vi "macro_MecaDrivePoseEst2_Execute.vi"() -> ()   [LabVIEW 2019, in "Trajectory_Library.lvlib"]
uses:
  Trajectory_Library.lvlib
  TypeDef/POSE2D.ctl
  TypeDef/TRANSLATION2D.ctl
  TypeDef/ROTATION2D.ctl
  TypeDef/MECA_WHEEL_POSITIONS.ctl
  VI/Util_GetTime_U32.vi
  VI/Util_GetTime_U64.vi
panel:
  in  "Wheel Distances":T1 {"RearRight" format="%19.3f"; "RearLeft" format="%19.3f"; "FrontRight" format="%19.3f"; "FrontLeft" format="%19.3f"}
  in  "Vision TImeStamp_Seconds":dbl=0.02
  in  "visionRobotPose":T2={"TRANSLATION"={"X"=0.0, "Y"=0.0}, "ROTATION"={"VALUE"=0.0, "COS"=1.0, "SIN"=0.0}} {"ROTATION"."SIN" format="%13.4f"; "ROTATION"."COS" format="%13.4f"; "ROTATION"."VALUE" format="%13.4f"; "TRANSLATION"."Y" format="%14.3f"; "TRANSLATION"."X" format="%14.3f"}
  in  "Add Vision Meas":bool
  in  "Game Started":bool=TRUE
  in  "InitialPose":T2={"TRANSLATION"={"X"=0.0, "Y"=0.0}, "ROTATION"={"VALUE"=0.0, "COS"=1.0, "SIN"=0.0}} {"ROTATION"."SIN" format="%13.4f"; "ROTATION"."COS" format="%13.4f"; "ROTATION"."VALUE" format="%13.4f"; "TRANSLATION"."Y" format="%14.3f"; "TRANSLATION"."X" format="%14.3f"}
  in  "Gyro Degrees":dbl
  out "Estimated Pose":T2={"TRANSLATION"={"X"=0.0, "Y"=0.0}, "ROTATION"={"VALUE"=0.0, "COS"=1.0, "SIN"=0.0}} {"ROTATION"."SIN" format="%13.4f"; "ROTATION"."COS" format="%13.4f"; "ROTATION"."VALUE" format="%13.4f"; "TRANSLATION"."Y" format="%14.3f"; "TRANSLATION"."X" format="%14.3f"}
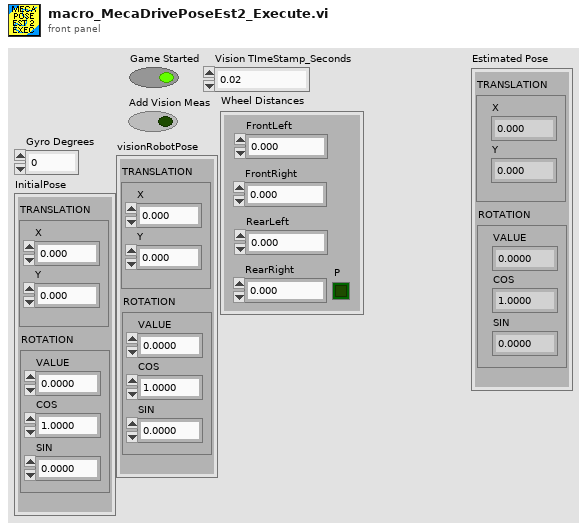
[diagram p1: front panel]
types:
  T1 = typedef "Trajectory_Library.lvlib/MECA_WHEEL_POSITIONS.ctl" = cluster{"FrontLeft":dbl, "FrontRight":dbl, "RearLeft":dbl, "RearRight":dbl, "P":bool}
  T2 = typedef "Trajectory_Library.lvlib/POSE2D.ctl" = cluster{"TRANSLATION":T3, "ROTATION":T4}
  T3 = typedef "Trajectory_Library.lvlib/TRANSLATION2D.ctl" = cluster{"X":dbl, "Y":dbl}
  T4 = typedef "Trajectory_Library.lvlib/ROTATION2D.ctl" = cluster{"VALUE":dbl, "COS":dbl, "SIN":dbl}
  T5 = typedef "Trajectory_Library.lvlib/MECA_DRIVE_POSE_EST2_CONFIG.ctl" = cluster{"Rear Left Wheel M":T3, "Odom X std dev M":dbl, "Odom Y std dev M":dbl, "Odom Heading std dev Rad":dbl, "Vision X std dev M":dbl, "Vision Y std dev M":dbl, "Vision Heading std dev Rad":dbl, "Front Left Wheel M":T3, "Front Right Wheel M":T3, "Rear Right Wheel M":T3}
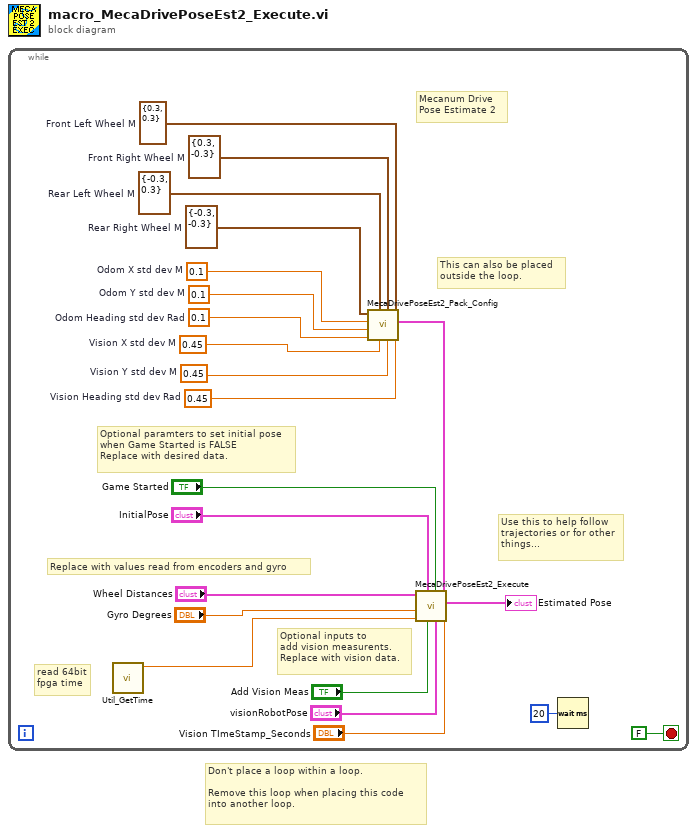
[diagram p0: block diagram]
diagram:
  # "Don't place a loop within a loop.\n \nRemove this loop when placing this code\ninto another loop."
  n1 = while {
    stop <- FALSE stop-if-true
    w1 = T3 {"X"=-0.3, "Y"=-0.3}  # Rear Right Wheel M
    w2 = T3 {"X"=-0.3, "Y"=0.3}  # Rear Left Wheel M
    w3 = T3 {"X"=0.3, "Y"=-0.3}  # Front Right Wheel M
    w4 = T3 {"X"=0.3, "Y"=0.3}  # Front Left Wheel M
    w15 = 0.1  # Odom Y std dev M
    w16 = 0.1  # Odom Heading std dev Rad
    w17 = 0.45  # Vision X std dev M
    w18 = 0.45  # Vision Y std dev M
    w19 = 0.1  # Odom X std dev M
    w20 = 0.45  # Vision Heading std dev Rad
    # "Optional inputs to\nadd vision measurents.\nReplace with vision data."
    # "Replace with values read from encoders and gyro"
    # "Optional paramters to set initial pose\nwhen Game Started is FALSE\nReplace with desired data."
    # "read 64bit\nfpga time"
    # "This can also be placed \noutside the loop."
    # "Use this to help follow\ntrajectories or for other\nthings..."
    # "Mecanum Drive \nPose Estimate 2"
    n2 = call "Util_GetTime.vi"() -> ("FPGA_Time_Seconds"=w12:dbl)  [unwired: 9 in, 2 out]
    n3 = call "MecaDrivePoseEst2_Pack_Config.vi"("Vision Heading std dev Rad"=w20, "Front Left Wheel M"=w4, "Vision Y std dev M"=w18, "Front Right Wheel M"=w3, "Vision X std dev M"=w17, "Rear Left Wheel M"=w2, "Odom Heading std dev Rad"=w16, "Odom Y std dev M"=w15, "Odom X std dev M"=w19, "Rear Right Wheel M"=w1) -> ("MecaPoseEst2Config"=w6:T5)  [unwired: 1 in]
    n4 = call "MecaDrivePoseEst2_Execute.vi"("Vision TImeStamp_Seconds"="Vision TImeStamp_Seconds", "MecaPoseEst2Config"=w6, "visionRobotPose"="visionRobotPose", "Game Started"="Game Started", "Add Vision Meas"="Add Vision Meas", "InitialPose"="InitialPose", "Pass Through Time"=w12, "Gyro Degrees"="Gyro Degrees", "Wheel Distances"="Wheel Distances") -> ("Estimated Pose"=→"Estimated Pose":T2)  [unwired: 1 in, 1 out]
    n5 = Wait (ms)(milliseconds to wait=u32 20) -> ()  [unwired: 1 out]
  }
